vi "Read Description.vi"(8 "error in (no error)":errorcluster, 11 "TAF Proj Document Type:FrontPanelGUI in":refnum<class "FrontPanelGUI.lvclass">) -> (0 "error out":errorcluster, 2 "Description":string, 3 "TAF Proj Document Type:FrontPanelGUI out":refnum<class "FrontPanelGUI.lvclass">)   [LabVIEW 2021]
uses:
  <vilib>/Wovalab/AntiDoc/Document Type/Add-ons/LabVIEW YAF Project/FrontPanelGUI/FrontPanelGUI.lvclass
  C:/Program Files (x86)/National Instruments/LabVIEW 2021/vi.lib/Wovalab/AntiDoc/Bloc/Bloc.lvclass
  C:/Program Files (x86)/National Instruments/LabVIEW 2021/vi.lib/Wovalab/AntiDoc/Document Type/Add-ons/LabVIEW YAF Project/FrontPanelGUI/FrontPanelGUI.lvclass
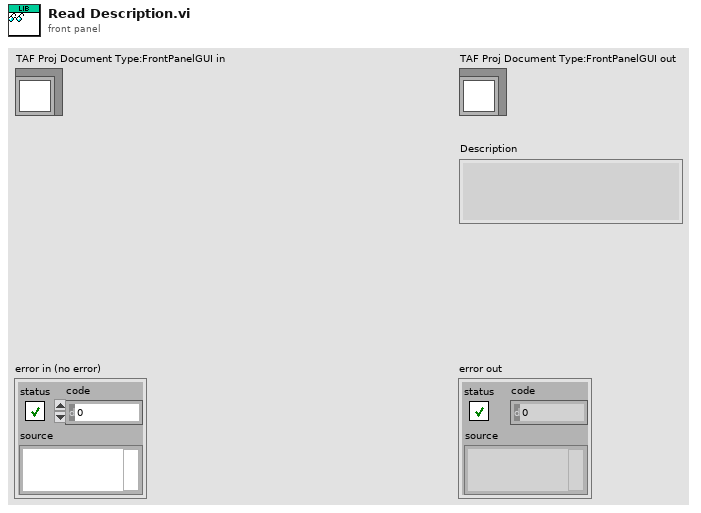
[diagram p1: front panel]
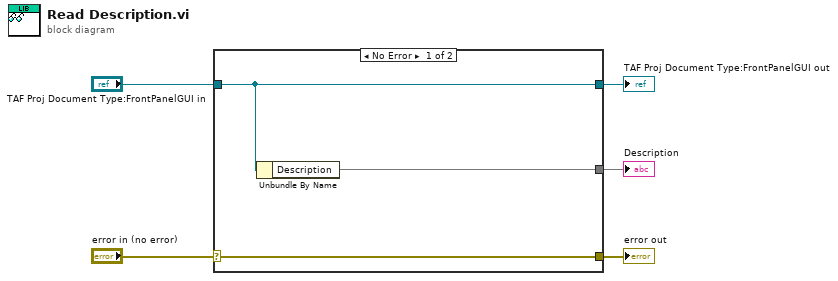
[diagram p0: block diagram]
diagram:
  n1 = case shown="No Error" "error in (no error)" {
    selector: "error in (no error)" -> [w8 w9]
    tunnel: [w8 w9] -> w4
    tunnel: [w7 w10] -> w2
    tunnel: "TAF Proj Document Type:FrontPanelGUI in" -> [w7 w10]
    tunnel: [w6 _] -> w1
    frame No Error {
      n2 = Unbundle By Name(w7) -> ("Description"=w6)
    }
    frame Error {
    }
  }
  "error out" <- w4
  "TAF Proj Document Type:FrontPanelGUI out" <- w2
  "Description" <- w1
